vi "Out of range.vi"(0 "Sensor Data":T1 {"Sensor array"."scaled" format="%.2f"; "Sensor array"."voltage" format="%.4f"; "Time" format="%<%I:%M:%S%2u %p\n%m/%d/%Y>T"}) -> (1 "Out of Range":bool)   [LabVIEW 2015]
uses:
  TCP DAQ/Sensor data.ctl
  DAQ configuration/sensor cluster.ctl
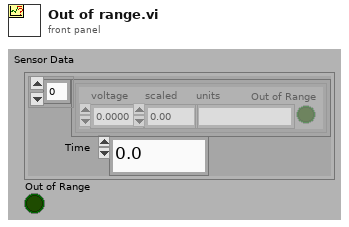
[diagram p1: front panel]
types:
  T1 = typedef "Sensor data.ctl" = cluster{" Sensor array":T2[], "Time":dbl}
  T2 = typedef "sensor cluster.ctl" = cluster{"voltage":sgl, "scaled":sgl, "units":string, "Out of Range":bool}
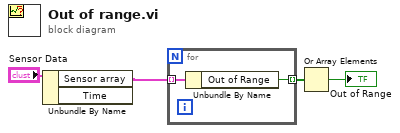
[diagram p0: block diagram]
diagram:
  n1 = Unbundle By Name("Sensor Data") -> ("Sensor array"=w3:T2[])  [unwired: 1 out]
  n2 = for {
    tunnel: w3 -> [w6] mode=indexing
    tunnel: [w5] -> w2 mode=indexing
    n3 = Unbundle By Name(w6) -> ("Out of Range"=w5:bool)
  }
  n4 = Or Array Elements(Boolean array=w2) -> (logical OR=→"Out of Range":bool)
